vi "WfLOfpaTester.vi"() -> ()   [LabVIEW 2013]
panel:
  in  "Delay (ms) In":i32=2000
  out "random (0 to 1)":dbl
  out "millisecond timer value":u32
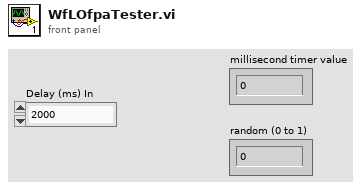
[diagram p1: front panel]
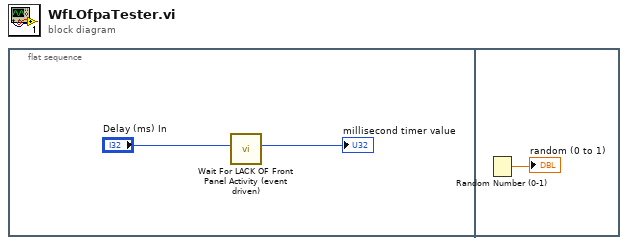
[diagram p0: block diagram]
diagram:
  n1 = flat-sequence {
    frame #0 {
      n2 = call <userlib>:"Wait For LACK OF Front Panel Activity (event driven).vi"("Minimum Wait Time (ms)"="Delay (ms) In") -> ("Actual Wait Time (ms)"=→"millisecond timer value":i64)  [unwired: 9 in]
    }
    frame #1 {
      n3 = Random Number (0-1)() -> (number: 0 to 1=→"random (0 to 1)":dbl)
    }
  }
